vi "Read TreeBar.vi"(8 "error in (no error)":errorcluster, 11 "BetterHandle in":refnum<class "BetterHandle.lvclass">) -> (0 "error out":errorcluster, 2 "Event Sequencer.lvlib:BetterTreeBar.lvclass":refnum<class "BetterHorizontalBar.lvclass">, 3 "BetterHandle out":refnum<class "BetterHandle.lvclass">)   [LabVIEW 2020, in "BetterDragAndDrop.lvlib" / "BetterHandle.lvclass"]
uses:
  BetterHandle.lvclass
  BetterTreeBar/BetterHorizontalBar.lvclass
  BetterHandle.lvclass/BetterHandle.ctl
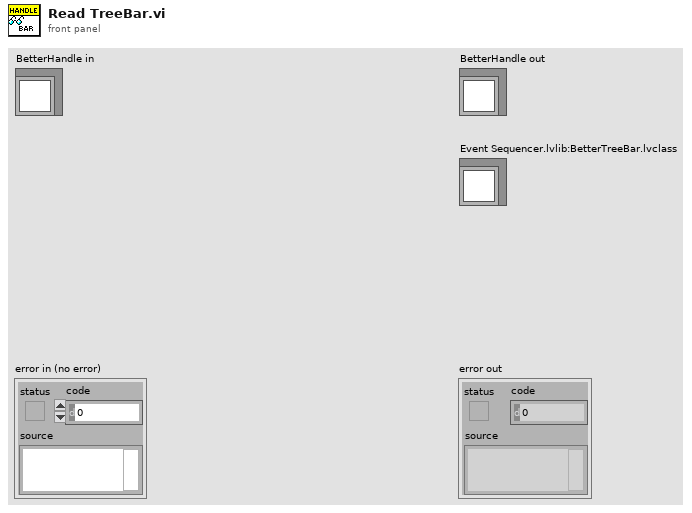
[diagram p1: front panel]
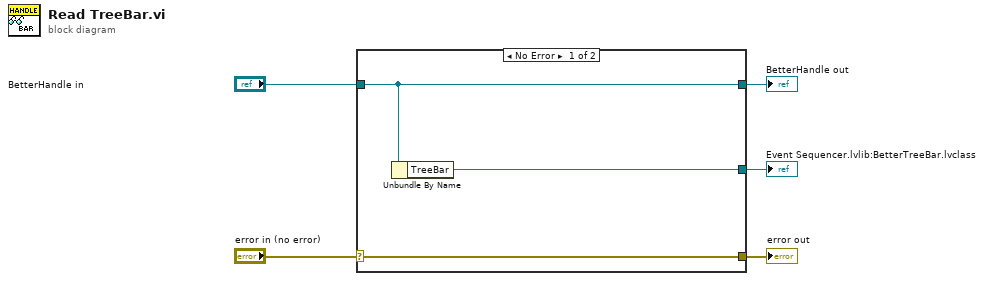
[diagram p0: block diagram]
diagram:
  n1 = case shown="No Error" "error in (no error)" {
    selector: "error in (no error)" -> [w8 w9]
    tunnel: [w8 w9] -> w4
    tunnel: [w7 w10] -> w2
    tunnel: "BetterHandle in" -> [w7 w10]
    tunnel: [w6 _] -> w1
    frame No Error {
      n2 = Unbundle By Name(w7) -> ("TreeBar"=w6:refnum<class "BetterHorizontalBar.lvclass">)
    }
    frame Error {
    }
  }
  "error out" <- w4
  "BetterHandle out" <- w2
  "Event Sequencer.lvlib:BetterTreeBar.lvclass" <- w1
